vi "mks946_sub_get.vi"(7 "mks946_comm":string="PR", 8 "error in (no error)":errorcluster, 9 "mks946_ch":u8, 10 "mks946_id":i32, 11 "VISA_ref_in":refnum<visa-resource-name>="COM3") -> (0 "error out":errorcluster={"status"=TRUE, "code"=1, "source"="Scan From String (arg 1) in mks946_sub_get.vi"}, 1 "Boolean":bool, 2 "mks946_res_def":T1, 3 "VISA_ref_out":refnum<visa-resource-name>="COM3")   [LabVIEW 2020]
uses:
  mks946_controls/ctrl_mks946_res.ctl
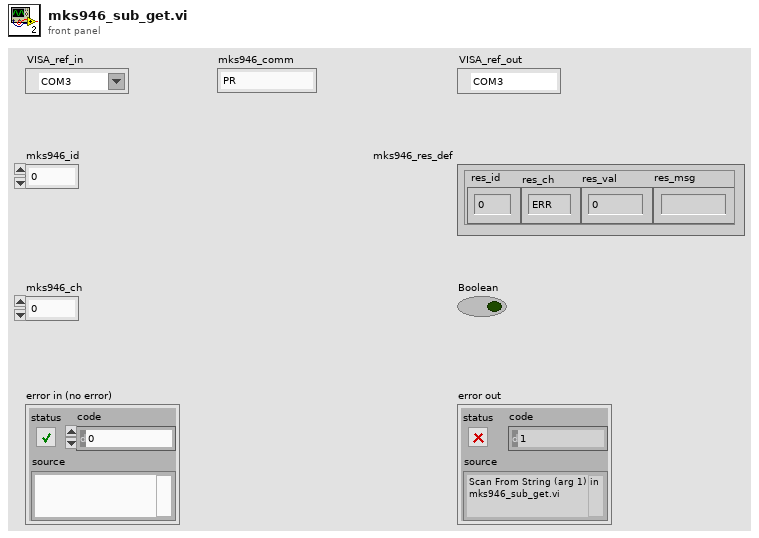
[diagram p1: front panel]
types:
  T1 = typedef "ctrl_mks946_res.ctl" = cluster{"res_ch":enum8{"ERR", "1", "2", "3", "4", "5", "6"}, "res_val":dbl, "res_id":u8, "res_msg":string}
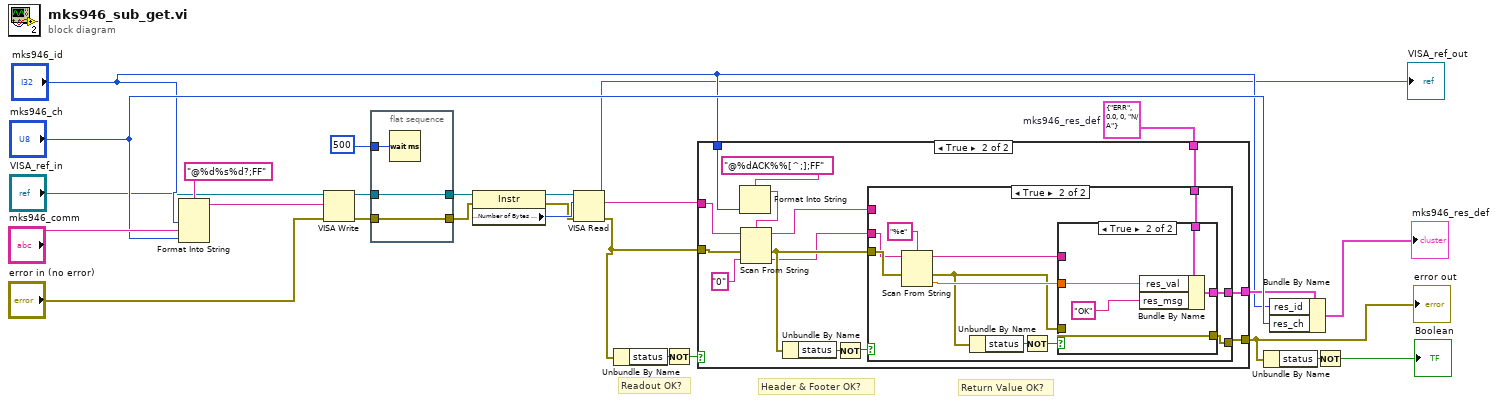
[diagram p0: block diagram]
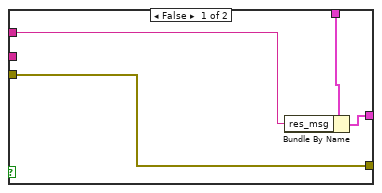
[diagram p3: hidden frame]
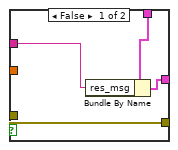
[diagram p4: hidden frame]
diagram:
  w23 = T1 {"res_ch"=enum."ERR", "res_val"=0.0, "res_id"=0, "res_msg"="N/A"}  # mks946_res_def
  # "Return Value OK?"
  # "Header & Footer OK?"
  # "Readout OK?"
  n1 = Format Into String(format string="@%d%s%d?;FF", "mks946_id", "mks946_comm", "mks946_ch") -> (resulting string=w6:string)  [unwired: 2 in, 1 out]
  n2 = VISA Write(VISA resource name="VISA_ref_in", write buffer=w6, error in (no error)="error in (no error)") -> (VISA resource name out=w2:refnum<visa-resource-name>, error out=w1:errorcluster)  [unwired: 1 out]
  n3 = flat-sequence {
    tunnel: w1 -> [w28]
    tunnel: [w28] -> w11
    tunnel: w2 -> [w27]
    tunnel: [w27] -> w10
    tunnel: u32 500 ("mks946_delay") -> [w29]
    frame #0 {
      n4 = Wait (ms)(milliseconds to wait=w29) -> ()  [unwired: 1 out]
    }
  }
  n5 = property class="Instr"(reference=w10, error in=w11) -> (reference out=w20:refnum<visa-resource-name>, error out=w21:errorcluster, "Serial Settings:Number of Bytes at Serial Port"=w22:u32)
  n6 = VISA Read(VISA resource name=w20, byte count=w22, error in (no error)=w21) -> (VISA resource name out=→"VISA_ref_out":refnum<visa-resource-name>, read buffer=w13:string, error out=w14:errorcluster)  [unwired: 1 out]
  n7 = Unbundle By Name(w14) -> ("status"=w9:bool)
  n8 = Not(x=w9) -> (.not. x?=w12:bool)
  n9 = case shown="True" w12 {
    tunnel: [w30 w34] -> w17
    tunnel: w23 -> [w31 w36]
    tunnel: [w31 w35] -> w19
    tunnel: w13 -> [_ w45]
    tunnel: w14 -> [w30 w44]
    tunnel: "mks946_id" -> [_ w43]
    frame False {
    }
    frame True {
      n10 = Format Into String(format string="@%dACK%%[^;];FF", w43) -> (resulting string=w42:string)  [unwired: 2 in, 1 out]
      n11 = Scan From String(format string=w42, input string=w45, error in=w44, default 1="0") -> (remaining string=w33:string, error out=w38:errorcluster, output 1=w37:string)  [unwired: 1 in, 1 out]
      n12 = Unbundle By Name(w38) -> ("status"=w40:bool)
      n13 = Not(x=w40) -> (.not. x?=w39:bool)
      n14 = case shown="True" w39 {
        tunnel: w38 -> [w49 w59]
        tunnel: w37 -> [_ w58]
        tunnel: w36 -> [w47 w56]
        tunnel: [w48 w54] -> w35
        tunnel: [w49 w51] -> w34
        tunnel: w33 -> [w46 _]
        frame False {
          n15 = Bundle By Name(cluster=w47, "res_msg"=w46) -> (w48:T1)
        }
        frame True {
          n16 = Scan From String(format string="%e", input string=w58, error in=w59) -> (remaining string=w50:string, error out=w52:errorcluster, output 1=w55:dbl)  [unwired: 2 in, 1 out]
          n17 = Unbundle By Name(w52) -> ("status"=w57:bool)
          n18 = Not(x=w57) -> (.not. x?=w53:bool)
          n19 = case shown="True" w53 {
            tunnel: w56 -> [w62 w69]
            tunnel: w55 -> [_ w68]
            tunnel: [w63 w66] -> w54
            tunnel: w52 -> [w64 w65]
            tunnel: [w64 w65] -> w51
            tunnel: w50 -> [w61 _]
            frame False {
              n20 = Bundle By Name(cluster=w62, "res_msg"=w61) -> (w63:T1)
            }
            frame True {
              n21 = Bundle By Name(cluster=w69, "res_val"=w68, "res_msg"="OK") -> (w66:T1)
            }
          }
        }
      }
    }
  }
  "error out" <- w17
  n22 = Unbundle By Name(w17) -> ("status"=w15:bool)
  n23 = Bundle By Name(cluster=w19, "res_id"="mks946_id", "res_ch"="mks946_ch") -> (→"mks946_res_def":T1)
  n24 = Not(x=w15) -> (.not. x?=→"Boolean":bool)
